vi "Test FTDI SPI Set Channel.vi"() -> ()   [LabVIEW 2018]
uses:
  PROJEKT/NIKO/Labview/Niko V4/FTDI SPI/Ctl/Sub Addr.ctl
panel:
  in  "nCS":u8 max=2 step=1
  out "handle out":u32
  in  "Mode":T1(ring)
  in  "Addr":T2 items=["Addr-0", "Addr-1", "Addr-2", "Addr-3", "Addr-4", "Addr-5", "Addr-6", "Addr-7"]
  out "LATCH Reg":u16
  in  "Channel Decimal":u16 max=10
  out "error out":errorcluster
  in  "Relays (1-10)":bool[](array[boolean])=[FALSE, FALSE, FALSE, FALSE, FALSE, FALSE, FALSE, FALSE, FALSE, FALSE]
  out "OK":bool
  out "Ini Status":bool
  in  "config":T3={"ClockRate"=50000, "LatencyTimer"=10, "configOptions 24-31"=0, "configOptions 16-23"=0, "configOptions 8-15"=0, "configOptions 0-7"=32, "Pin"=0, "reserved"=0} {"configOptions 24-31" format="%x"; "configOptions 16-23" format="%x"; "configOptions 8-15" format="%x"; "configOptions 0-7" format="%x"}
  # "configOptions\nThis member provides a way to enable/disable features\n\tspecific to the protocol that are implemented in the chip\n\tBIT1-0=CPOL-CPHA:\t00 - MODE0 - data captured on rising edge, propagated on falling\n \t\t\t\t\t\t01 - MODE1 - data captured on falling edge, propagated on rising\n \t\t\t\t\t\t10 - MODE2 - data captured on falling edge, propagated on rising\n \t\t\t\t\t\t11 - MODE3 - data captured on rising edge, propagated on falling\n\tBIT4-BIT2: 000 - A/B/C/D_DBUS3=ChipSelect\n\t\t\t : 001 - A/B/C/D_DBUS4=ChipSelect\n \t\t\t : 010 - A/B/C/D_DBUS5=ChipSelect\n \t\t\t : 011 - A/B/C/D_DBUS6=ChipSelect\n \t\t\t : 100 - A/B/C/D_DBUS7=ChipSelect\n \tBIT5: ChipSelect is active high if this bit is 0\n\tBIT6 -BIT31\t\t: Reserved"
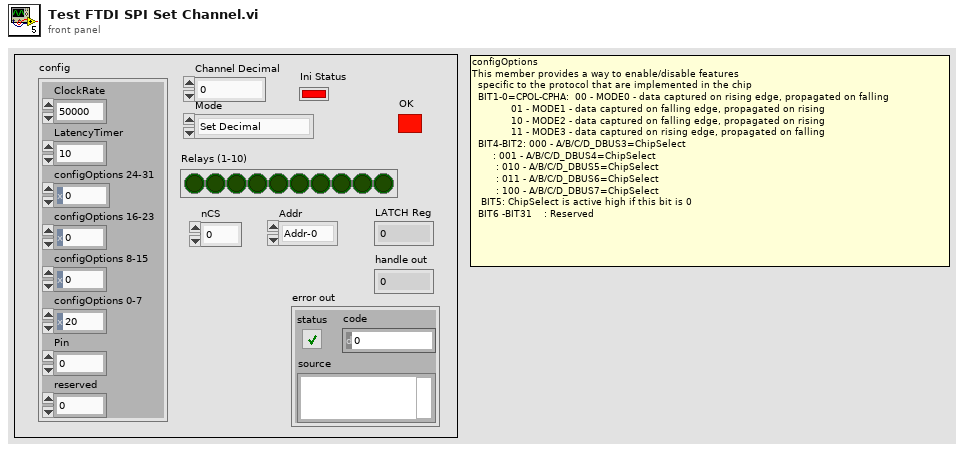
[diagram p1: front panel]
types:
  T1 = enum16{"Set Decimal", "Set Binary", "Set Channels", "Reset Channels", "Togle Channel"}
  T2 = typedef "Sub Addr.ctl" = u16
  T3 = cluster{"ClockRate":u32, "LatencyTimer":u8, "configOptions 24-31":i8, "configOptions 16-23":i8, "configOptions 8-15":i8, "configOptions 0-7":u32, "Pin":u32, "reserved":u16}
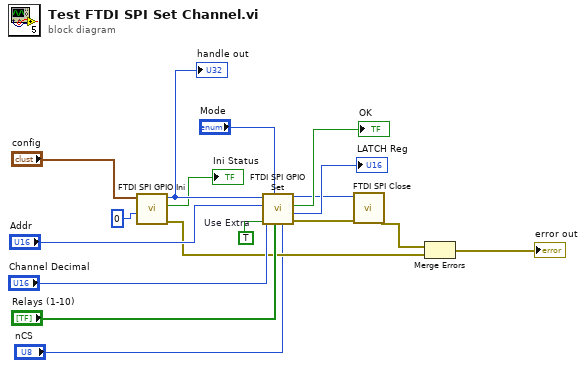
[diagram p0: block diagram]
diagram:
  w13 = TRUE  # Use Extra
  n1 = call "FTDI SPI GPIO Ini.vi"("Channel Nmb"=u8 0 ("FTDI Dev Nmb"), "config"="config") -> ("error out"=w7:errorcluster, "Ini Status"=→"Ini Status":bool, "handle out"=w9:u32)  [unwired: 5 in, 2 out]
  "handle out" <- w9
  n2 = call "FTDI SPI GPIO Set.vi"("nCS"="nCS", "Relays (1-10)"="Relays (1-10)", "Mode"="Mode", "Use Extra"=w13, "Channel Decimal"="Channel Decimal", "Addr"="Addr", "Handler In"=w9) -> ("error out"=w6:errorcluster, "LATCH Reg"=→"LATCH Reg":u16, "OK"=→"OK":bool, "Handler Out"=w5:u32)  [unwired: 1 in]
  n3 = call "FTDI SPI Close.vi"("error in (no error)"=w6, "Handler In"=w5) -> ("error out"=w4:errorcluster)  [unwired: 9 in]
  n4 = Merge Errors(w4, w7) -> (→"error out":errorcluster)
